vi "Exercise 3-1 with loop.vi"() -> ()   [LabVIEW 2014]
panel:
  out "Warning?":bool
  out "Warning Text":string
  in  "Min Temp":dbl
  in  "Max Temp":dbl
  in  "Current Temp":dbl
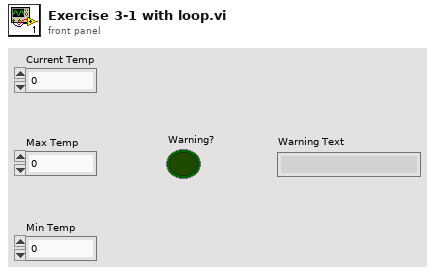
[diagram p1: front panel]
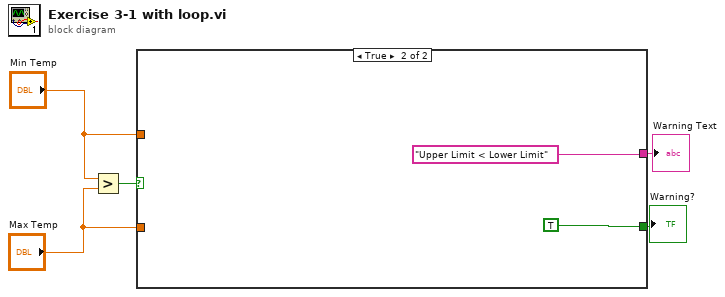
[diagram p0: block diagram]
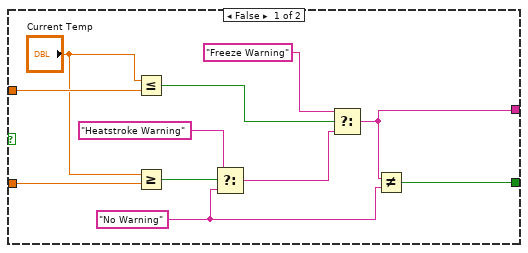
[diagram p2: hidden frame]
diagram:
  n1 = Greater?(x="Min Temp", y="Max Temp") -> (0:w5:bool)
  n2 = case shown="True" w5 {
    tunnel: "Min Temp" -> [w15 _]
    tunnel: "Max Temp" -> [w16 _]
    tunnel: [w9 "Upper Limit < Lower Limit"] -> w2
    tunnel: [w8 TRUE] -> w1
    frame False {
      w10 = "No Warning"
      n3 = Less Or Equal?(x="Current Temp", y=w15) -> (x <= y?=w13:bool)
      n4 = Greater Or Equal?(x="Current Temp", y=w16) -> (x >= y?=w11:bool)
      n5 = Select(t="Heatstroke Warning", s=w11, f=w10) -> (s? t:f=w7:string)
      n6 = Select(t="Freeze Warning", s=w13, f=w7) -> (s? t:f=w9:string)
      n7 = Not Equal?(x=w9, y=w10) -> (x != y?=w8:bool)
    }
    frame True {
    }
  }
  "Warning Text" <- w2
  "Warning?" <- w1
